vi "testWarning.vi"() -> ()   [LabVIEW 2019, in "AssertionTest.lvlib" / "AssertNoError.lvlib"]
uses:
  AssertNoError.lvlib
  <vilib>/Utility/error.llb/Error Cluster From Error Code.vi
  <vilib>/ErrorRing/Error Ring.xnode
  Assertion/Assertion.lvlib
panel:
  out "error out":errorcluster
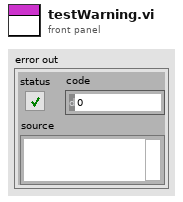
[diagram p1: front panel]
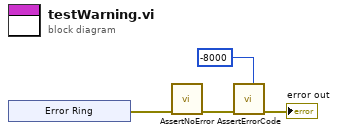
[diagram p0: block diagram]
diagram:
  n1 = xnode "Error Ring"() -> ("error out"=w4:errorcluster)
  n2 = call "AssertNoError.vi"("error in (no error)"=w4) -> ("error out"=w1:errorcluster)  [unwired: 10 in]
  n3 = call "AssertErrorCode.vi"("Expected"=-8000, "error in (no error)"=w1) -> ("error out"=→"error out":errorcluster)  [unwired: 9 in]
